vi "NI VeriStand - Open Percent Complete Notification.vi"(8 "error in (no error)":errorcluster, 11 "MacroPlayer in":T2) -> (0 "error out":errorcluster, 2 "PercentComplete Refs":T1, 3 "MacroPlayer out":T2)   [LabVIEW 2020, in "NI_VS MacroPlayerAPI.lvlib"]
doc: "Opens a reference to messages the Macro Player sends that indicate the percentage of the macro file that has played back. This VI returns a user event that you can register and wire to an Event structure."
uses:
  <vilib>/NI VeriStand/Execution/MacroPlayer/NI_VS MacroPlayerAPI.lvlib
  <vilib>/NI VeriStand/Execution/MacroPlayer/MacroPlayerAPI.ctl
  NationalInstruments.VeriStand.ClientAPI
  <vilib>/NI VeriStand/Execution/MacroPlayer/PercentComplete Refs.ctl
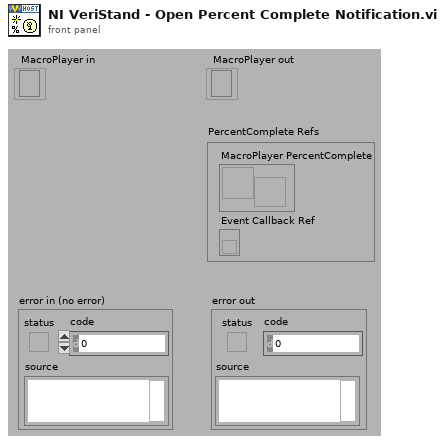
[diagram p1: front panel]
types:
  T1 = typedef "NI_VS MacroPlayerAPI.lvlib/PercentComplete Refs.ctl" = cluster{"MacroPlayer PercentComplete":refnum<user-event>, "Event Callback Ref":refnum<k27>}
  T2 = typedef "NI_VS MacroPlayerAPI.lvlib/MacroPlayerAPI.ctl" = refnum<k24>
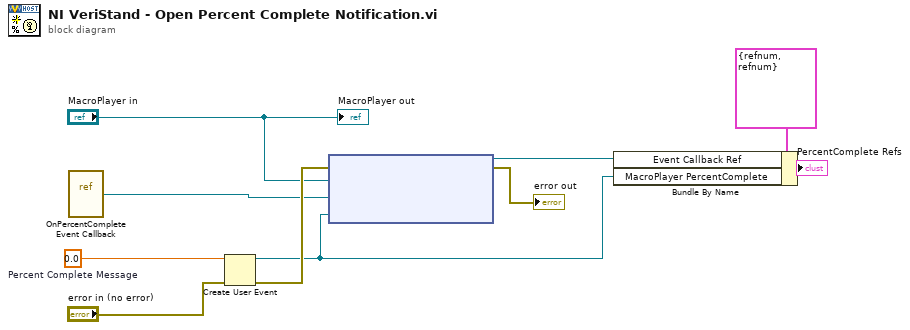
[diagram p0: block diagram]
diagram:
  w10 = 0.0  # Percent Complete Message
  n1 = vi-ref <vilib>:"OnPercentComplete Event Callback.vi"() -> ("vi reference"=w3:refnum<vi>)
  n2 = Create User Event(user event datatype=w10, error in="error in (no error)") -> (user event=w2:refnum<user-event>, error out=w9:errorcluster)
  n3 = node(w9, "MacroPlayer in", w3, w2) -> (w5:refnum<k27>, →"error out":errorcluster)  [unwired: 1 in]
  n4 = Bundle By Name(cluster=T1 {"MacroPlayer PercentComplete"=refnum, "Event Callback Ref"=refnum} ("Percent Complete Refs"), "Event Callback Ref"=w5, "MacroPlayer PercentComplete"=w2) -> (→"PercentComplete Refs":T1)
  "MacroPlayer out" <- "MacroPlayer in"
